vi "Building Automation Assignment.vi"() -> ()   [LabVIEW 2017]
panel:
  out "AC ON OFF":bool
  out "Numeric Indicator":dbl
  out "Solar Power Details":dynamicdata(graph)
  in  "Switch to Solar":bool
  in  "Battery Level Sensor":dbl(slide) scale=0.0..10.0
  in  "Remove Button":bool
  in  "Add Button":bool
  in  "Room Temp Sensor":dbl(slide) scale=0.0..100.0
  in  "Fire Sensor":bool
  in  "Water Meter":dbl
  out "EM 2":dbl
  out "EM":dbl
  in  "Electric Meter":dbl
  in  "Door PIR sensor":bool
  out "Light Level":dbl(slide) scale=0.0..100.0
  in  "Garden Light Sensor":dbl(slide) scale=0.0..100.0
  in  "Stair case PIR sensor":bool
  out "Main Power":bool
  out "Solar Power":bool
  out "Battery Level":dbl(knob) scale=0.0..10.0
  in  "EME":bool
  out "Fire light":bool
  in  "A/C ON - OFF":bool
  out "Room Temp (C)":dbl(slide) scale=0.0..100.0
  in  "Auto - Manual 2":bool
  out "Door":bool
  in  "Manual Switch":bool
  in  "Auto - Manual":bool
  in  "Auto - Manual":bool
  out "Garden Light":bool
  in  "Manual Switch":bool
  out "Stair Case Light":bool
  in  "Manual Switch":bool
  # "Automatic  Staircase Lights"
  # "Air Cooling System"
  # "Solar Power Controlling"
  # "`C"
  # "Temperture"
  # "Automatic Garden Light"
  # "Fire Alarm Controlling"
  # "Electric Meter"
  # "Water Meter"
  # "Motion Sensitive Door"
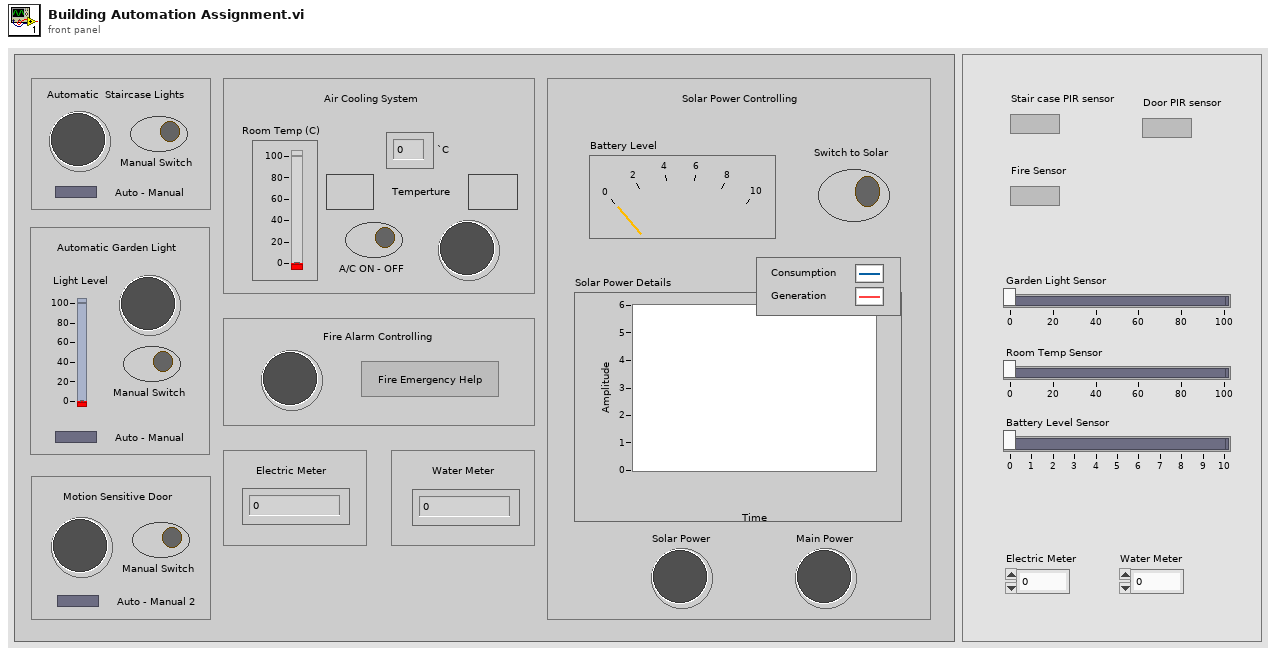
[diagram p1: front panel]
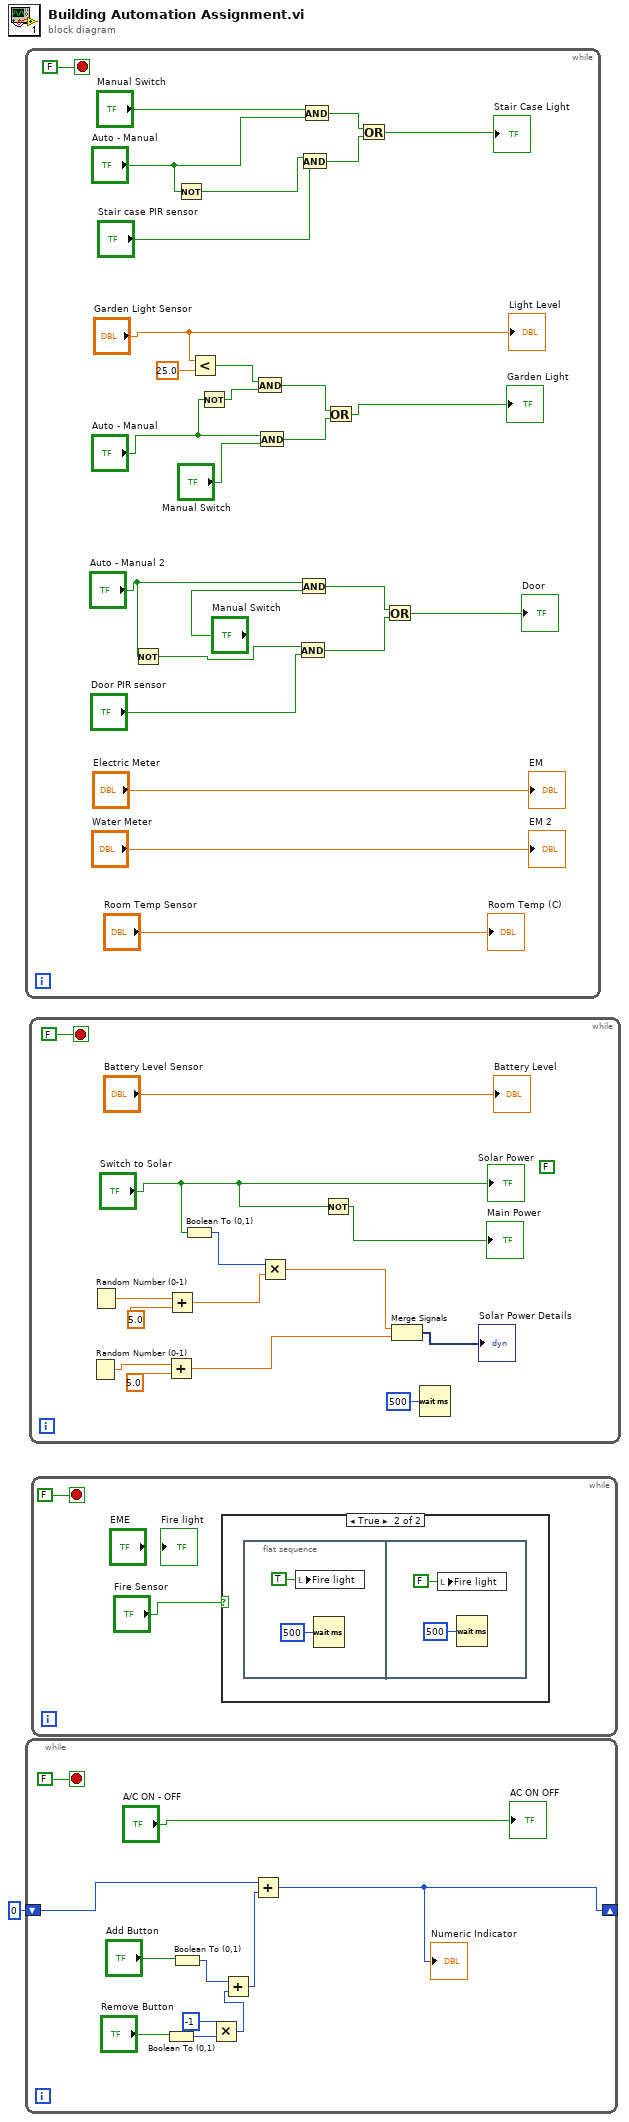
[diagram p0: block diagram]
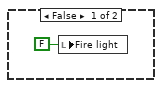
[diagram p2: hidden frame]
diagram:
  n1 = while {
    stop <- FALSE stop-if-true
    n2 = Not(x="Auto - Manual 2") -> (.not. x?=w10:bool)
    n3 = Not(x="Auto - Manual") -> (.not. x?=w27:bool)
    n4 = Less?(x="Garden Light Sensor", y=25.0) -> (x < y?=w18:bool)
    n5 = Not(x="Auto - Manual") -> (.not. x?=w16:bool)
    n6 = And(x=w18, y=w16) -> (x .and. y?=w15:bool)
    n7 = And(x="Auto - Manual", y="Manual Switch") -> (x .and. y?=w14:bool)
    n8 = And(x=w10, y="Door PIR sensor") -> (x .and. y?=w7:bool)
    n9 = And(x="Auto - Manual 2", y="Manual Switch") -> (x .and. y?=w8:bool)
    n10 = And(x=w27, y="Stair case PIR sensor") -> (x .and. y?=w24:bool)
    n11 = And(x="Manual Switch", y="Auto - Manual") -> (x .and. y?=w25:bool)
    n12 = Or(x=w15, y=w14) -> (x .or. y?=→"Garden Light":bool)
    n13 = Or(x=w25, y=w24) -> (x .or. y?=→"Stair Case Light":bool)
    n14 = Or(x=w8, y=w7) -> (x .or. y?=→"Door":bool)
    "Light Level" <- "Garden Light Sensor"
    "EM" <- "Electric Meter"
    "EM 2" <- "Water Meter"
    "Room Temp (C)" <- "Room Temp Sensor"
  }
  n15 = while {
    shift-right: [w36] -> _
    shift-left: 0 -> [w38]
    stop <- FALSE stop-if-true
    n16 = Boolean To (0,1)(Boolean="Remove Button") -> (0, 1=w32:i16)
    n17 = Boolean To (0,1)(Boolean="Add Button") -> (0, 1=w35:i16)
    n18 = Multiply(x=i16 -1, y=w32) -> (x*y=w30:i16)
    n19 = Add(x=w35, y=w30) -> (x+y=w34:i16)
    n20 = Add(x=w38, y=w34) -> (x+y=w36:i32)
    "Numeric Indicator" <- w36
    "AC ON OFF" <- "A/C ON - OFF"
  }
  n21 = while {
    stop <- FALSE stop-if-true
    (unwired) FALSE
    n22 = Random Number (0-1)() -> (number: 0 to 1=w47:dbl)
    n23 = Random Number (0-1)() -> (number: 0 to 1=w46:dbl)
    n24 = Add(x=w47, y=5.0) -> (x+y=w48:dbl)
    n25 = Add(x=w46, y=5.0) -> (x+y=w52:dbl)
    n26 = Boolean To (0,1)(Boolean="Switch to Solar") -> (0, 1=w51:i16)
    n27 = Multiply(x=w51, y=w52) -> (x*y=w53:dbl)
    n28 = Not(x="Switch to Solar") -> (.not. x?=→"Main Power":bool)
    n29 = Merge Signals(w53, w48) -> (→"Solar Power Details":dynamicdata)
    n30 = Wait (ms)(milliseconds to wait=u32 500) -> ()  [unwired: 1 out]
    "Solar Power" <- "Switch to Solar"
    "Battery Level" <- "Battery Level Sensor"
  }
  n31 = while {
    stop <- FALSE stop-if-true
    n32 = case shown="True" "Fire Sensor" {
      frame False {
        n33 = local write "Fire light"(FALSE ("Fire light")) -> ()
      }
      frame True {
        n34 = flat-sequence {
          frame #0 {
            n35 = local write "Fire light"(TRUE ("Fire light")) -> ()
            n36 = Wait (ms)(milliseconds to wait=u32 500) -> ()  [unwired: 1 out]
          }
          frame #1 {
            n37 = local write "Fire light"(FALSE ("Fire light")) -> ()
            n38 = Wait (ms)(milliseconds to wait=u32 500) -> ()  [unwired: 1 out]
          }
        }
      }
    }
  }
